vi "lm Init.vi"(8 "error in (no error)":errorcluster, 10 "LETypeStr":string, 11 "ComPort":i32) -> (0 "error out":errorcluster, 2 "LETypeStr out":string, 3 "function return":u32)   [LabVIEW 2017, in "LumencorDLLDbg64.lvlib"]
doc: "Initializes the Selected LE on the Com port specified. Sets all Color Levels to zero and the enables to OFF.\n\n\nextern \"C\" LUMENCORDLL2B_API HANDLE lmInit(int ComPort, char *LETypeStr);"
uses:
  LumencorDLLDbg64.lvlib
  LumencorDLLDbg64.dll
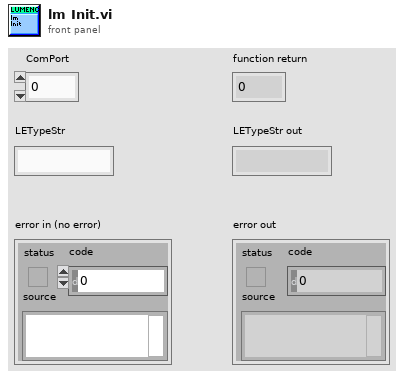
[diagram p1: front panel]
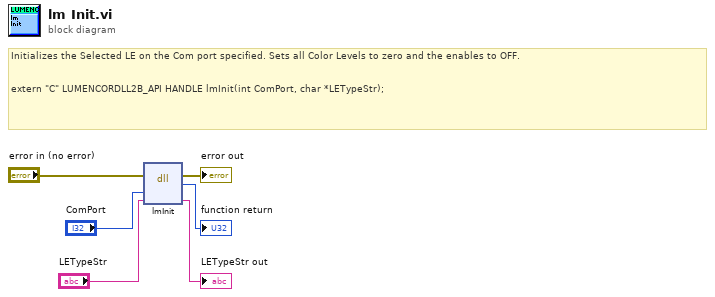
[diagram p0: block diagram]
diagram:
  # "Initializes the Selected LE on the Com port specified. Sets all Color Levels to zero and the enables to OFF.\n\n\nextern \"C\" LUMENCORDLL2B_API HANDLE lmInit(int ComPort, char *LETypeStr);"
  n1 = dll-call lib="Q:/GIT -- Lumencor DLL4/LabVIEW Library (64bit)/LumencorDLLDbg64.*" fn="lmInit"(error in="error in (no error)", "ComPort"="ComPort", "LETypeStr"="LETypeStr") -> (error out=→"error out":errorcluster, →"function return":u32, "LETypeStr"=→"LETypeStr out":string)  [unwired: 3 in, 1 out]
